vi "SetDataSourceFingerprint.vi"(8 "error in":errorcluster, 10 "DataSourceFingerprint":string, 11 "Datawarehouse in":refnum<class "Datawarehouse.lvclass">) -> (0 "error out":errorcluster, 3 "Datawarehouse out":refnum<class "Datawarehouse.lvclass">)   [LabVIEW 2021, in "ProligentXMLGenerator.lvlib" / "Datawarehouse.lvclass"]
doc: "The information contained in this attribute is used to protect the data warehouse from the\ninjection of the same file more than once. The rule is that all files that contain the\nsame fingerprint as a file that has already been processed successfully by the DIT will\nbe rejected.\n\nFor example, if the file contains information about a product unit, a good value for the\nfingerprint would be the product unit serial number followed by the generation date of the\nXSD.\n\nIf the attribute is ommited, the DIT will generate a random fingerprint. The result is\nthat it will now be possible to inject the same file more than once.\n\nThis value is limited to 448 charactesrs and must no be empty."
uses:
  Datawarehouse.lvclass
  Datawarehouse.lvclass/Datawarehouse.ctl
  Base/NonEmptyString_448/NonEmptyString_448.lvclass
  Base/Attribute/Attribute.lvclass
  C:/Projects/proligent-xml-generator-labview/src/ProligentXMLGenerator/Base/NonEmptyString/NonEmptyString.lvclass
  C:/Projects/proligent-xml-generator-labview/src/ProligentXMLGenerator/Base/String/String.lvclass
  C:/Projects/proligent-xml-generator-labview/src/ProligentXMLGenerator/Base/Attribute/Attribute.lvclass
  C:/Projects/proligent-xml-generator-labview/src/ProligentXMLGenerator/Base/NonEmptyString_448/NonEmptyString_448.lvclass
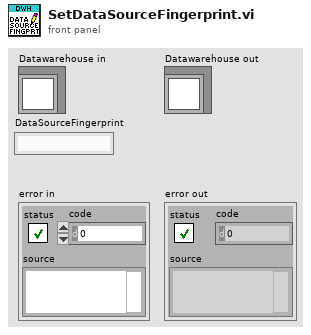
[diagram p1: front panel]
types:
  T1 = typedef "ProligentXMLGenerator.lvlib/Datawarehouse.lvclass/Data.ctl" = cluster{"DestinationFolder":path, "BaseFileName":string, "Document":refnum<k20>, "Defects":refnum<class "Defect.lvclass">[], "TopProcessRuns":refnum<class "ProcessRun.lvclass">[], "ProductUnits":refnum<class "ProductUnit.lvclass">[], "GenerationTime":refnum<class "DateTime.lvclass">, "DataSourceFingerprint":refnum<class "NonEmptyString_448.lvclass">, "IntegrationMetaData":refnum<class "NonEmptyString_2000.lvclass">, "TimeZoneInfoId":string}
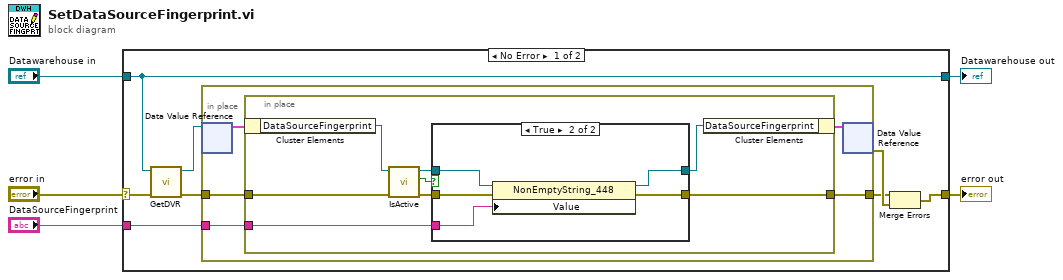
[diagram p0: block diagram]
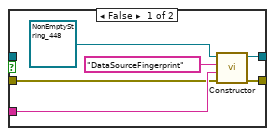
[diagram p2: hidden frame]
diagram:
  n1 = case shown="No Error" "error in" {
    selector: "error in" -> [w11 w38]
    tunnel: "Datawarehouse in" -> [w6 w39]
    tunnel: [w8 w38] -> w3
    tunnel: "DataSourceFingerprint" -> [w7 _]
    tunnel: [w6 w39] -> w1
    frame No Error {
      n2 = call "GetDVR.vi"("error in"=w11, "Datawarehouse"=w6) -> ("error out"=w10:errorcluster, "DVRReference"=w12:refnum<data-value>)  [unwired: 8 in]
      n3 = in-place "In Place Element Structure" {
        in-place-border: w10 -> [w16]
        in-place-border: [w18] -> w9
        in-place-border: w7 -> [w17]
        n4 = in-place-dvr #1(w12) -> (w15:T1)  [unwired: 1 out]
        n5 = in-place "In Place Element Structure" {
          in-place-border: [w26] -> w18
          in-place-border: w17 -> [w25]
          in-place-border: w16 -> [w24]
          n6 = in-place-cluster #2(w15) -> ("DataSourceFingerprint"=w20:refnum<class "NonEmptyString_448.lvclass">)
          n7 = call "IsActive.vi"("error in"=w24, "Attribute in"=w20) -> ("error out"=w21:errorcluster, "IsActive"=w22:bool, "Attribute in"=w23:refnum<class "NonEmptyString_448.lvclass">)  [unwired: 7 in]
          n8 = case shown="True" w22 {
            tunnel: [w29 w37] -> w26
            tunnel: w25 -> [w31 w33]
            tunnel: w23 -> [_ w36]
            tunnel: w21 -> [w30 w35]
            tunnel: [w27 w34] -> w19
            frame False {
              n9 = call-dynamic "Constructor.vi"("error in"=w30, "Value"=w31, "Name"="DataSourceFingerprint", "String in"=refnum<class "NonEmptyString_448.lvclass"> refnum ("ProligentCanonicalFile:NonEmptyString_448")) -> ("error out"=w29:errorcluster, "String out"=w27:refnum<class "NonEmptyString_448.lvclass">)  [unwired: 6 in]
            }
            frame True {
              n10 = property on="Property Node" class="NonEmptyString_448"(reference=w36, error in=w35, "Value"=w33) -> (reference out=w34:refnum<class "NonEmptyString_448.lvclass">, error out=w37:errorcluster)
            }
          }
          n11 = in-place-cluster #2("DataSourceFingerprint"=w19) -> (w14:T1)
        }
        n12 = in-place-dvr #1(w14) -> (w13:errorcluster)  [unwired: 1 out]
      }
      n13 = Merge Errors(w9, w13) -> (w8:errorcluster)
    }
    frame Error {
    }
  }
  "error out" <- w3
  "Datawarehouse out" <- w1
